vi "Reset.vi"(8 "error in":errorcluster, 11 "host in":refnum<class "LIA Host Interface FPGA.lvclass">) -> (0 "error out":errorcluster, 3 "host out":refnum<class "LIA Host Interface FPGA.lvclass">)   [LabVIEW 2018, in "LIA Host Interface FPGA.lvclass"]
uses:
  LIA Host Interface FPGA.lvclass
  Properties/FpgaSession_GET.vi
  host/Lock-In Amplifier Example Host.lvlib
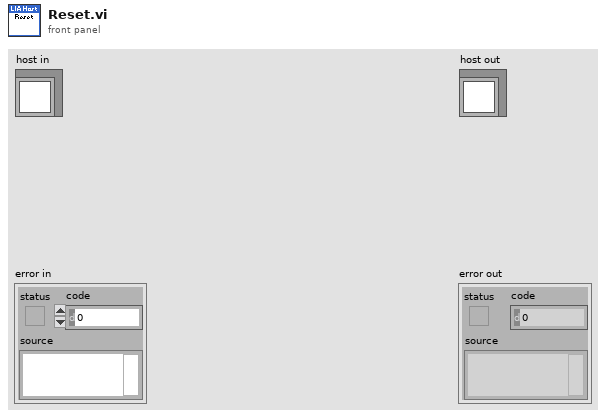
[diagram p1: front panel]
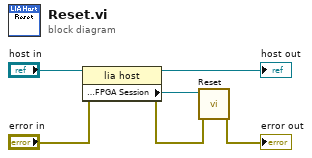
[diagram p0: block diagram]
diagram:
  n1 = property class="lia host"(reference="host in", error in="error in") -> (reference out=→"host out":refnum<class "LIA Host Interface FPGA.lvclass">, error out=w1:errorcluster, "Properties:FPGA Session"=w3:refnum<k20>)
  n2 = call "Reset.vi"("error in"=w1, "fpga session in"=w3) -> ("error out"=→"error out":errorcluster)  [unwired: 8 in, 1 out]
